vi "LinearFilter_HighPass.vi"(9 "SamplePeriod":dbl format="%13.5p", 11 "TimeConstant":dbl format="%13.5p") -> (3 "LINEAR_FILTER":T1 {"Outputs" format="%13.5g"; "Inputs" format="%13.5g"; "OutputGains" format="%13.5g"; "InputGains" format="%13.5g"})   [LabVIEW 2019, in "Trajectory_Library.lvlib"]
doc: "Creates a first-order high-pass filter of the form: \n\n y[n] = gain*x[n] + (-gain)*x[n-1] + gain*y[n-1] \n\n where \n\n gain = e^(-dt / T), \n T is the time constant in seconds.\n \nThis filter is stable for time constants greater than zero.\n \nInputs:\n - timeConstant The discrete-time time constant in seconds.\n - samplePeriod The period in seconds between samples taken by the user.\n \nOutputs:\n - Linearfilter - Created datat structure"
uses:
  Trajectory_Library.lvlib
  TypeDef/LINEAR_FILTER.ctl
  <vilib>/Rock Robotics/SystemInterfaces/NetworkCommunication/NetComm_UsageReport_report.vi
  Globals/Util_LibraryGlobals.vi
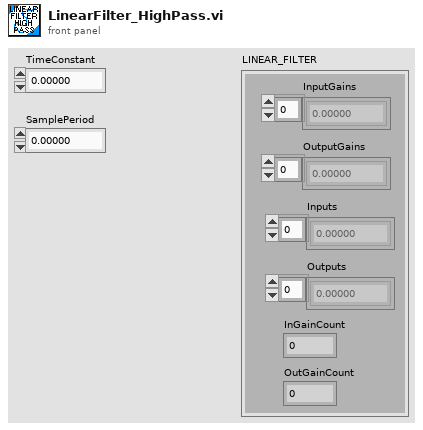
[diagram p1: front panel]
types:
  T1 = typedef "Trajectory_Library.lvlib/LINEAR_FILTER.ctl" = cluster{"InputGains":dbl[], "OutputGains":dbl[], "Inputs":dbl[], "Outputs":dbl[], "InGainCount":i32, "OutGainCount":i32}
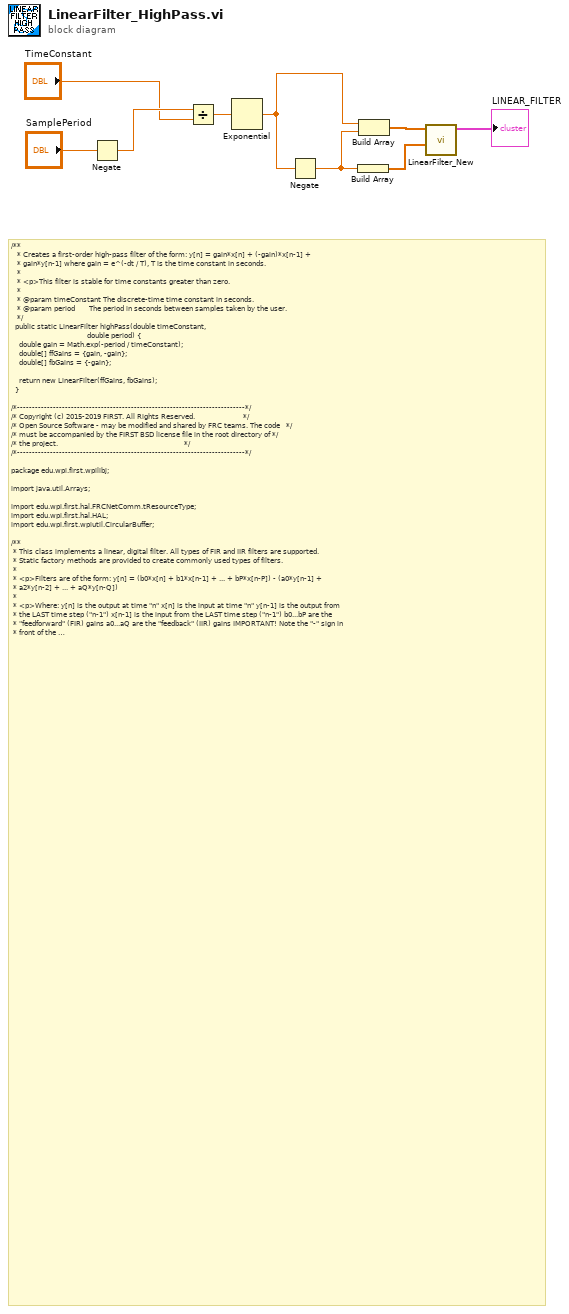
[diagram p0: block diagram]
diagram:
  # "/**\n   * Creates a first-order high-pass filter of the form: y[n] = gain*x[n] + (-gain)*x[n-1] +\n   * gain*y[n-1] where gain = e^(-dt / T), T is the time constant in seconds.\n   *\n   * <p>This filter is stable for time constants greater than zero.\n   *\n   * @param timeConstant The discrete-time time constant in seconds.\n   * @param period       The period in seconds between samples taken by the user.\n   */\n  public static LinearFilter highPass(double timeConstant,\n                                      double period) {\n    double gain = Math.exp(-period / timeConstant);\n    double[] ffGains = {gain, -gain};\n    double[] fbGains = {-gain};\n\n    return new LinearFilter(ffGains, fbGains);\n  }\n\n/*----------------------------------------------------------------------------*/\n/* Copyright (c) 2015-2019 FIRST. All Rights Reserved.                        */\n/* Open Source Software - may be modified and shared by FRC teams. The code   */\n/* must be accompanied by the FIRST BSD license file in the root directory of */\n/* the project.                                                               */\n/*----------------------------------------------------------------------------*/\n\npackage edu.wpi.first.wpilibj;\n\nimport java.util.Arrays;\n\nimport edu.wpi.first.hal.FRCNetComm.tResourceType;\nimport edu.wpi.first.hal.HAL;\nimport edu.wpi.first.wpiutil.CircularBuffer;\n\n/**\n * This class implements a linear, digital filter. All types of FIR and IIR filters are supported.\n * Static factory methods are provided to create commonly used types of filters.\n *\n * <p>Filters are of the form: y[n] = (b0*x[n] + b1*x[n-1] + ... + bP*x[n-P]) - (a0*y[n-1] +\n * a2*y[n-2] + ... + aQ*y[n-Q])\n *\n * <p>Where: y[n] is the output at time \"n\" x[n] is the input at time \"n\" y[n-1] is the output from\n * the LAST time step (\"n-1\") x[n-1] is the input from the LAST time step (\"n-1\") b0...bP are the\n * \"feedforward\" (FIR) gains a0...aQ are the \"feedback\" (IIR) gains IMPORTANT! Note the \"-\" sign in\n * front of the feedback term! This is a common convention in signal processing.\n *\n * <p>What can linear filters do? Basically, they can filter, or diminish, the effects of\n * undesirable input frequencies. High frequencies, or rapid changes, can be indicative of sensor\n * noise or be otherwise undesirable. A \"low pass\" filter smooths out the signal, reducing the\n * impact of these high frequency components.  Likewise, a \"high pass\" filter gets rid of\n * slow-moving signal components, letting you detect large changes more easily.\n *\n * <p>Example FRC applications of filters: - Getting rid of noise from an analog sensor input (note:\n * the roboRIO's FPGA can do this faster in hardware) - Smoothing out joystick input to prevent the\n * wheels from slipping or the robot from tipping - Smoothing motor commands so that unnecessary\n * strain isn't put on electrical or mechanical components - If you use clever gains, you can make a\n * PID controller out of this class!\n *\n * <p>For more on filters, we highly recommend the following articles:<br>\n * https://en.wikipedia.org/wiki/Linear_filter<br>\n * https://en.wikipedia.org/wiki/Iir_filter<br>\n * https://en.wikipedia.org/wiki/Fir_filter<br>\n *\n * <p>Note 1: calculate() should be called by the user on a known, regular period. You can use a\n * Notifier for this or do it \"inline\" with code in a periodic function.\n *\n * <p>Note 2: For ALL filters, gains are necessarily a function of frequency. If you make a filter\n * that works well for you at, say, 100Hz, you will most definitely need to adjust the gains if you\n * then want to run it at 200Hz! Combining this with Note 1 - the impetus is on YOU as a developer\n * to make sure calculate() gets called at the desired, constant frequency!\n */"
  n1 = Negate(x="SamplePeriod") -> (-x=w9:dbl)
  n2 = Divide(x=w9, y="TimeConstant") -> (x/y=w8:dbl)
  n3 = Exponential(1:w8) -> (0:w2:dbl)
  n4 = Negate(x=w2) -> (-x=w1:dbl)
  n5 = Build Array(w1) -> (w6:dbl[])
  n6 = Build Array(w2, w1) -> (w7:dbl[])
  n7 = call "LinearFilter_New.vi"("OutputGains"=w6, "InputGains"=w7) -> ("LINEAR_FILTER"=→"LINEAR_FILTER":T1)  [unwired: 9 in]
